vi "MovCorrFuncs.vi"(7 "MovCorrFunc":T5(ring), 11 "Image":T3(plugin-control)) -> (3 "Reference Screen":T3(plugin-control))   [LabVIEW 2020]
uses:
  <vilib>/vision/Image Controls.llb/IMAQ Image.ctl
  <vilib>/vision/NI_Vision_Development_Module.lvlib
panel:
  out "Lines":T1(array[cluster]) {"End Point"."Y" format="%.2f"; "End Point"."X" format="%.2f"; "Start Point"."Y" format="%.2f"; "Start Point"."X" format="%.2f"}
  out "Number of Matches Returned":i32
  out "width":dbl
  out "height":dbl
  out "most Verital":T2
  out "most horizontal":T2
  out "got copy":bool=TRUE
  in  "LUT1":cluster{u16, u16}(slide)={0, 4095} caption="Slide" scale=0.0..4095.0
  out "Reference Rectangles":dbl[][](array[numeric]) format="%.2f"
  out "upper":u16
  out "lower":u16
  out "Number \nof Particles":i32
  out "Mean Value":sgl format="%.2f"
  out "Histogram Graph":T4 {"Incremental Value" format="%.2f"; "Starting Value" format="%.2f"}
  out "temp copy":T3
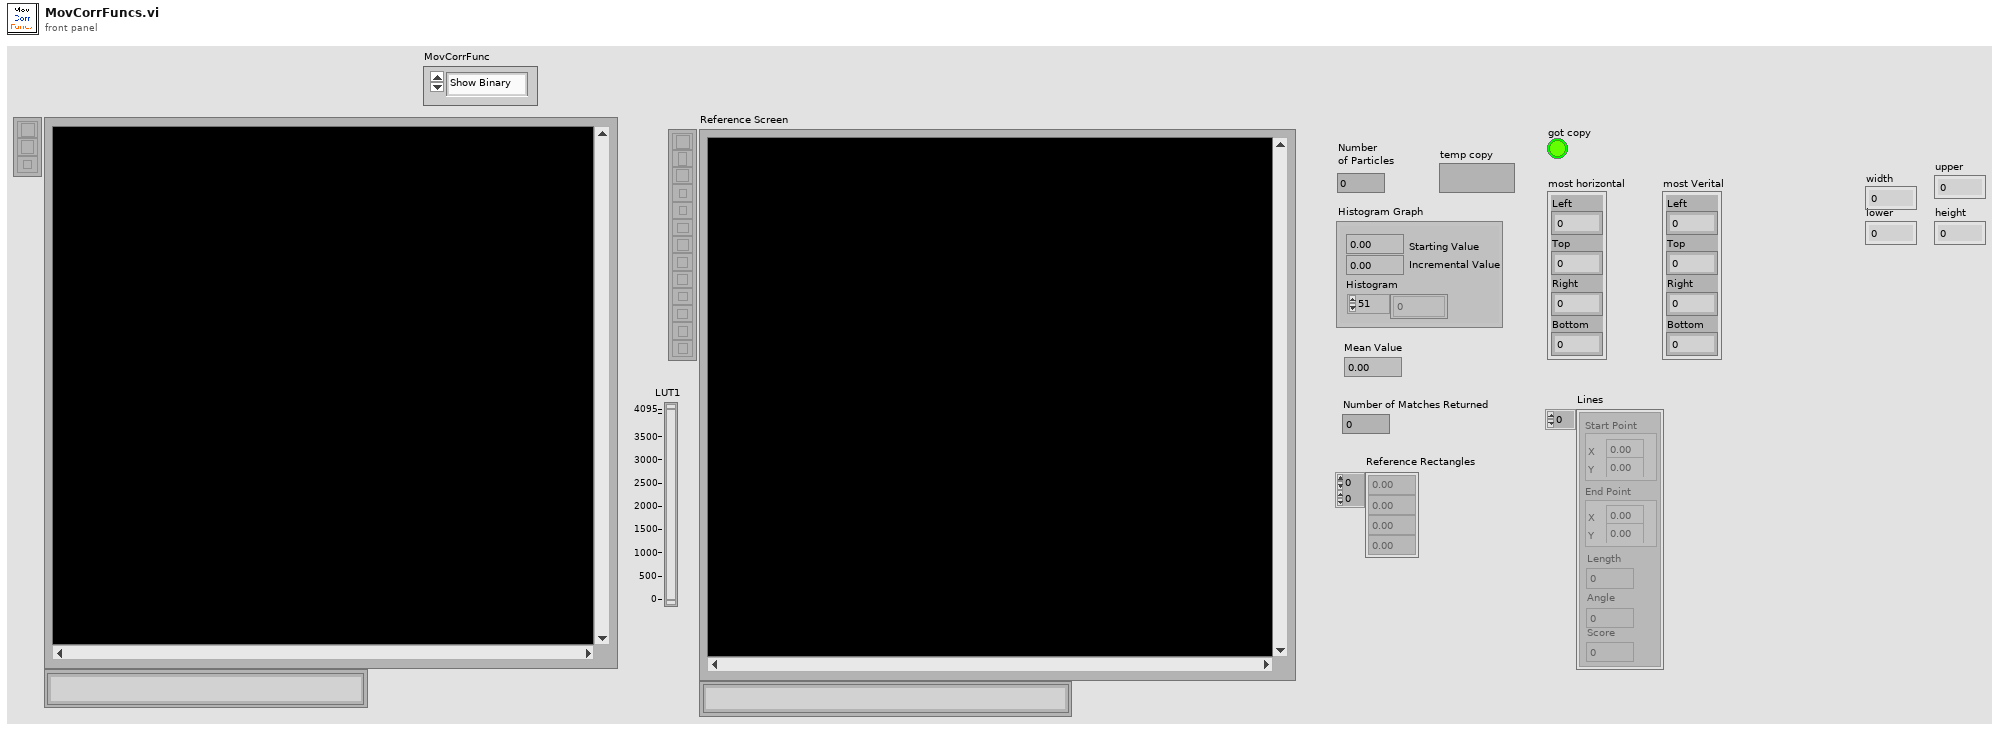
[diagram p1: front panel]
types:
  T1 = cluster{"Start Point":cluster{"X":sgl, "Y":sgl}, "End Point":cluster{"X":sgl, "Y":sgl}, "Length":dbl, "Angle":dbl, "Score":dbl}[]
  T2 = cluster{"Left":i32, "Top":i32, "Right":i32, "Bottom":i32}
  T3 = typedef "IMAQ Image.ctl" = refnum<image>
  T4 = cluster{"Starting Value":sgl, "Incremental Value":sgl, "Histogram":u32[]}
  T5 = enum16{"Show Binary", "Show Dendrite", "Find Lines"}
  T6 = enum32{"AutoM", "Close", "Dilate", "Erode", "Gradient", "Gradient out", "Gradient in", "Hit miss", "Open", "PClose", "POpen", "Thick", "Thin"}
  T7 = typedef "Particle Parameters" = i32
  T8 = typedef "Image Type" = u32
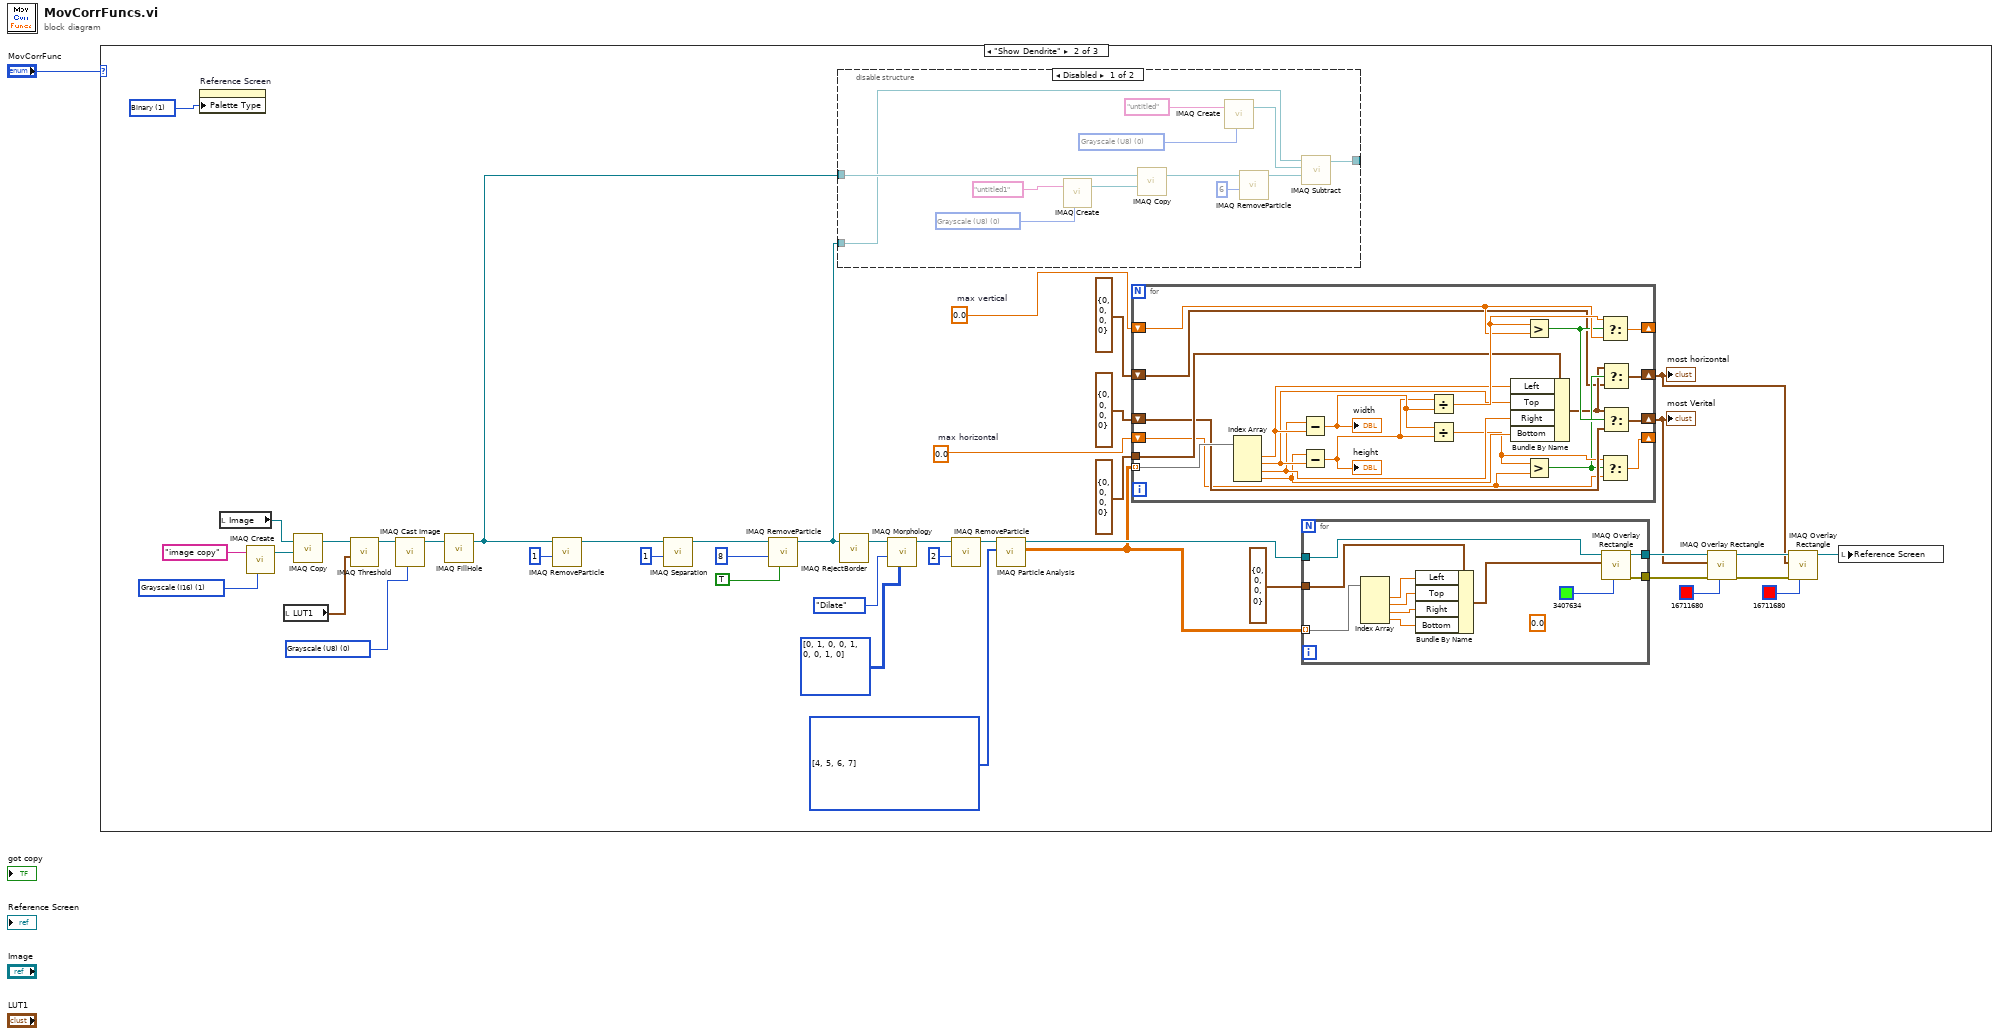
[diagram p0: block diagram]
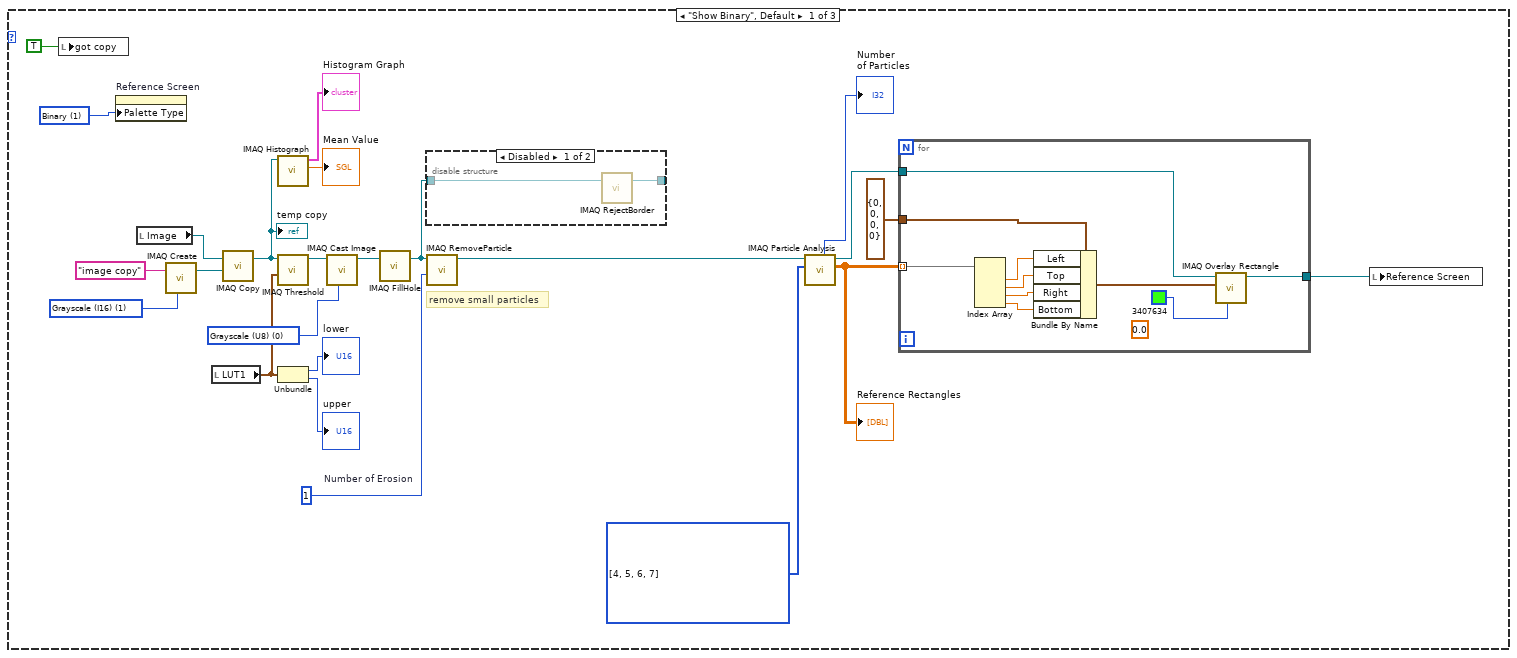
[diagram p2: hidden frame]
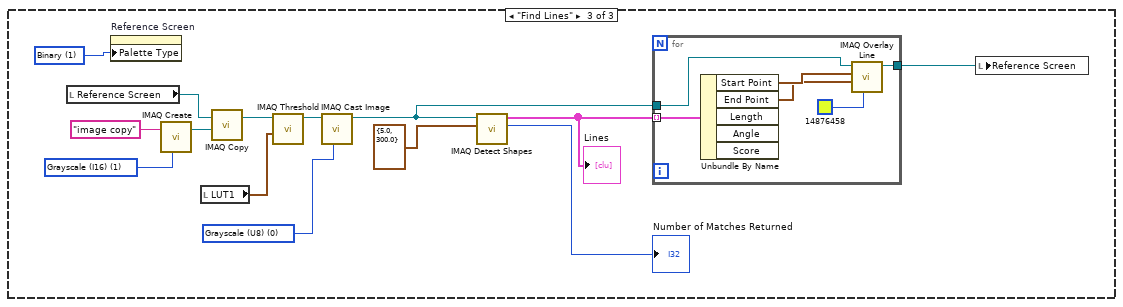
[diagram p5: hidden frame]
diagram:
  n1 = case shown="\"Show Dendrite\"" "MovCorrFunc" {
    frame "Show Binary", Default {
      w3 = u32 1 items=["Grayscale", "Binary", "Gradient", "Rainbow", "Temperature", "User Defined"] ("Palette:Palette Type")
      w12 = T7[] [4, 5, 6, 7] items=["Center of Mass X", "Center of Mass Y", "First Pixel X", "First Pixel Y", "Bounding Rect Left", "Bounding Rect Top", "Bounding Rect Right", "Bounding Rect Bottom", "Max Feret Diameter Start X", "Max Feret Diameter Start Y", "Max Feret Diameter End X", "Max Feret Diameter End Y", "Max Horiz. Segment Length Left", "Max Horiz. Segment Length Right", "Max Horiz. Segment Length Row", "-", "Bounding Rect Width", "Bounding Rect Height", "Bounding Rect Diagonal", "Perimeter", "Convex Hull Perimeter", "Holes' Perimeter", "Max Feret Diameter", "Equivalent Ellipse Major Axis", "Equivalent Ellipse Minor Axis", "Equivalent Ellipse Minor Axis (Feret)", "Equivalent Rect Long Side", "Equivalent Rect Short Side", "Equivalent Rect Diagonal", "Equivalent Rect Short Side (Feret)", "Average Horiz. Segment Length", "Average Vert. Segment Length", "Hydraulic Radius", "Waddel Disk Diameter", "-", "Area", "Holes' Area", "Particle & Holes' Area", "Convex Hull Area", "Image Area", "-", "Number of Holes", "Number of Horiz. Segments", "Number of Vert. Segments", "-", "Orientation", "Max Feret Diameter Orientation", "-", "% Area/Image Area", "% Area/(Particle & Holes' Area)", "Ratio of Equivalent Ellipse Axes", "Ratio of Equivalent Rect Sides", "-", "Elongation Factor", "Compactness Factor", "Heywood Circularity Factor", "Type Factor", "-", "Sum X", "Sum Y", "Sum XX", "Sum XY", "Sum YY", "Sum XXX", "Sum XXY", "Sum XYY", "Sum YYY", "-", "Moment of Inertia XX", "Moment of Inertia XY", "Moment of Inertia YY", "Moment of Inertia XXX", "Moment of Inertia XXY", "Moment of Inertia XYY", "Moment of Inertia YYY", "Norm. Moment of Inertia XX", "Norm. Moment of Inertia XY", "Norm. Moment of Inertia YY", "Norm. Moment of Inertia XXX", "Norm. Moment of Inertia XXY", "Norm. Moment of Inertia XYY", "Norm. Moment of Inertia YYY", "Hu Moment 1", "Hu Moment 2", "Hu Moment 3", "Hu Moment 4", "Hu Moment 5", "Hu Moment 6", "Hu Moment 7"] ("Pixel Measurements")
      w13 = 1  # Number of Erosion
      w15 = T8 0 items=["Grayscale (U8)", "Grayscale (I16)", "Grayscale (SGL)", "Complex (CSG)", "RGB (U32)", "HSL (U32)", "RGB (U64)", "Grayscale (U16)"] ("Image Type")
      w24 = T8 1 items=["Grayscale (U8)", "Grayscale (I16)", "Grayscale (SGL)", "Complex (CSG)", "RGB (U32)", "HSL (U32)", "RGB (U64)", "Grayscale (U16)"] ("Image Type")
      # "remove small particles"
      n2 = local write "got copy"(TRUE) -> ()
      n3 = property on="Reference Screen" class="ImageControl"("Palette Type"=w3) -> ()  [unwired: 2 in, 2 out]
      n4 = local read "Image"() -> (w19:T3)
      n5 = call "IMAQ Create"("Image Name"="image copy", "Image Type"=w24) -> ("New Image"=w23:T3)  [unwired: 3 in, 1 out]
      n6 = local read "LUT1"() -> (w14:cluster{u16, u16})
      n7 = call "IMAQ Copy"("Image Dst"=w23, "Image Src"=w19) -> ("Image Dst Out"=w18:T3)  [unwired: 4 in, 1 out]
      "temp copy" <- w18
      n8 = call "IMAQ Histograph"("Image"=w18) -> ("Mean Value"=→"Mean Value":sgl, "Histogram Graph"=→"Histogram Graph":T4)  [unwired: 7 in, 2 out]
      n9 = call "IMAQ Threshold"("Range"=w14, "Image Src"=w18) -> ("Image Dst Out"=w17:T3)  [unwired: 4 in, 5 out]
      n10 = Unbundle(w14) -> (→"lower":u16, →"upper":u16)
      n11 = call "IMAQ Cast Image"("Image Type"=w15, "Image Src"=w17) -> ("Image Dst Out"=w16:T3)  [unwired: 8 in, 1 out]
      n12 = call "IMAQ FillHole"("Image Src"=w16) -> ("Image Dst Out"=w2:T3)  [unwired: 3 in, 3 out]
      n13 = disable-structure shown="Disabled" {
        disable-tunnel: w2 -> [w27 _]
        disable-tunnel: [w26 _] -> _
        frame Disabled {
          n14 = call "IMAQ RejectBorder"("Image Src"=w27) -> ("Image Dst Out"=w26:T3)  [unwired: 3 in, 3 out]
        }
        frame Enabled {
        }
      }
      n15 = call "IMAQ RemoveParticle"("Number of Erosion"=w13, "Image Src"=w2) -> ("Image Dst Out"=w9:T3)  [unwired: 5 in, 4 out]
      n16 = call "IMAQ Particle Analysis"("Pixel Measurements"=w12, "Image"=w9) -> ("Particle Measurements (Pixels)"=w4:dbl[][], "Image Out (duplicate)"=w11:T3, "Number of Particles"=→"Number \nof Particles":i32)  [unwired: 4 in, 3 out]
      "Reference Rectangles" <- w4
      n17 = for {
        tunnel: [w28] -> w5
        tunnel: w11 -> [w36]
        tunnel: w4 -> [w34] mode=indexing
        tunnel: T2 {"Left"=0, "Top"=0, "Right"=0, "Bottom"=0} ("Rectangle") -> [w35]
        (unwired) 0.0 ("Rotation")
        n18 = Index Array(array=w34) -> (element #1=w32:dbl, element #2=w31:dbl, element #3=w30:dbl, element #4=w29:dbl)  [unwired: 4 in]
        n19 = Bundle By Name(cluster=w35, "Left"=w32, "Top"=w31, "Right"=w30, "Bottom"=w29) -> (w33:T2)
        n20 = call "IMAQ Overlay Rectangle"("Color"=u32 3407634 ("Text Color (black)"), "Rectangle"=w33, "Image"=w36) -> ("Image Out"=w28:T3)  [unwired: 7 in, 1 out]
      }
      n21 = local write "Reference Screen"(w5) -> ()
    }
    frame "Show Dendrite" {
      w53 = 0.0  # max horizontal
      w54 = 0.0  # max vertical
      w70 = T7[] [4, 5, 6, 7] items=["Center of Mass X", "Center of Mass Y", "First Pixel X", "First Pixel Y", "Bounding Rect Left", "Bounding Rect Top", "Bounding Rect Right", "Bounding Rect Bottom", "Max Feret Diameter Start X", "Max Feret Diameter Start Y", "Max Feret Diameter End X", "Max Feret Diameter End Y", "Max Horiz. Segment Length Left", "Max Horiz. Segment Length Right", "Max Horiz. Segment Length Row", "-", "Bounding Rect Width", "Bounding Rect Height", "Bounding Rect Diagonal", "Perimeter", "Convex Hull Perimeter", "Holes' Perimeter", "Max Feret Diameter", "Equivalent Ellipse Major Axis", "Equivalent Ellipse Minor Axis", "Equivalent Ellipse Minor Axis (Feret)", "Equivalent Rect Long Side", "Equivalent Rect Short Side", "Equivalent Rect Diagonal", "Equivalent Rect Short Side (Feret)", "Average Horiz. Segment Length", "Average Vert. Segment Length", "Hydraulic Radius", "Waddel Disk Diameter", "-", "Area", "Holes' Area", "Particle & Holes' Area", "Convex Hull Area", "Image Area", "-", "Number of Holes", "Number of Horiz. Segments", "Number of Vert. Segments", "-", "Orientation", "Max Feret Diameter Orientation", "-", "% Area/Image Area", "% Area/(Particle & Holes' Area)", "Ratio of Equivalent Ellipse Axes", "Ratio of Equivalent Rect Sides", "-", "Elongation Factor", "Compactness Factor", "Heywood Circularity Factor", "Type Factor", "-", "Sum X", "Sum Y", "Sum XX", "Sum XY", "Sum YY", "Sum XXX", "Sum XXY", "Sum XYY", "Sum YYY", "-", "Moment of Inertia XX", "Moment of Inertia XY", "Moment of Inertia YY", "Moment of Inertia XXX", "Moment of Inertia XXY", "Moment of Inertia XYY", "Moment of Inertia YYY", "Norm. Moment of Inertia XX", "Norm. Moment of Inertia XY", "Norm. Moment of Inertia YY", "Norm. Moment of Inertia XXX", "Norm. Moment of Inertia XXY", "Norm. Moment of Inertia XYY", "Norm. Moment of Inertia YYY", "Hu Moment 1", "Hu Moment 2", "Hu Moment 3", "Hu Moment 4", "Hu Moment 5", "Hu Moment 6", "Hu Moment 7"] ("Pixel Measurements")
      w72 = T8 0 items=["Grayscale (U8)", "Grayscale (I16)", "Grayscale (SGL)", "Complex (CSG)", "RGB (U32)", "HSL (U32)", "RGB (U64)", "Grayscale (U16)"] ("Image Type")
      w73 = u32 1 items=["Grayscale", "Binary", "Gradient", "Rainbow", "Temperature", "User Defined"] ("Palette:Palette Type")
      w78 = T8 1 items=["Grayscale (U8)", "Grayscale (I16)", "Grayscale (SGL)", "Complex (CSG)", "RGB (U32)", "HSL (U32)", "RGB (U64)", "Grayscale (U16)"] ("Image Type")
      n22 = property on="Reference Screen" class="ImageControl"("Palette Type"=w73) -> ()  [unwired: 2 in, 2 out]
      n23 = local read "Image"() -> (w76:T3)
      n24 = call "IMAQ Create"("Image Name"="image copy", "Image Type"=w78) -> ("New Image"=w77:T3)  [unwired: 3 in, 1 out]
      n25 = local read "LUT1"() -> (w74:cluster{u16, u16})
      n26 = call "IMAQ Copy"("Image Dst"=w77, "Image Src"=w76) -> ("Image Dst Out"=w75:T3)  [unwired: 4 in, 1 out]
      n27 = call "IMAQ Threshold"("Range"=w74, "Image Src"=w75) -> ("Image Dst Out"=w40:T3)  [unwired: 4 in, 5 out]
      n28 = call "IMAQ Cast Image"("Image Type"=w72, "Image Src"=w40) -> ("Image Dst Out"=w39:T3)  [unwired: 8 in, 1 out]
      n29 = call "IMAQ FillHole"("Image Src"=w39) -> ("Image Dst Out"=w38:T3)  [unwired: 5 in, 1 out]
      n30 = call "IMAQ RemoveParticle"("Number of Erosion"=1, "Image Src"=w38) -> ("Image Dst Out"=w67:T3)  [unwired: 5 in, 4 out]
      n31 = call "IMAQ Separation"("Nb of Erosion"=1, "Image Src"=w67) -> ("Image Dst Out"=w64:T3)  [unwired: 8 in, 1 out]
      n32 = call "IMAQ RemoveParticle"("Low Pass/High Pass (Low)"=TRUE, "Number of Erosion"=8, "Image Src"=w64) -> ("Image Dst Out"=w62:T3)  [unwired: 4 in, 4 out]
      n33 = disable-structure shown="Disabled" {
        disable-tunnel: w38 -> [w112 _]
        disable-tunnel: w62 -> [w111 _]
        disable-tunnel: [w110 _] -> _
        frame Disabled {
          w103 = T8 0 items=["Grayscale (U8)", "Grayscale (I16)", "Grayscale (SGL)", "Complex (CSG)", "RGB (U32)", "HSL (U32)", "RGB (U64)", "Grayscale (U16)"] ("Image Type")
          w108 = T8 0 items=["Grayscale (U8)", "Grayscale (I16)", "Grayscale (SGL)", "Complex (CSG)", "RGB (U32)", "HSL (U32)", "RGB (U64)", "Grayscale (U16)"] ("Image Type")
          n34 = call "IMAQ Create"("Image Name"="untitled1", "Image Type"=w103) -> ("New Image"=w102:T3)  [unwired: 3 in, 1 out]
          n35 = call "IMAQ Copy"("Image Dst"=w102, "Image Src"=w112) -> ("Image Dst Out"=w101:T3)  [unwired: 4 in, 1 out]
          n36 = call "IMAQ Create"("Image Name"="untitled", "Image Type"=w108) -> ("New Image"=w106:T3)  [unwired: 3 in, 1 out]
          n37 = call "IMAQ RemoveParticle"("Number of Erosion"=6, "Image Src"=w101) -> ("Image Dst Out"=w105:T3)  [unwired: 5 in, 4 out]
          n38 = call "IMAQ Subtract"("Image Src A"=w111, "Image Dst"=w106, "Image Src B"=w105) -> ("Image Dst Out"=w110:T3)  [unwired: 4 in, 1 out]
        }
        frame Enabled {
        }
      }
      n39 = call "IMAQ RejectBorder"("Image Src"=w62) -> ("Image Dst Out"=w60:T3)  [unwired: 5 in, 1 out]
      n40 = call "IMAQ Morphology"("Structuring Element"=i32[][] [[0, 1, 0], [0, 1, 0], [0, 1, 0]], "Operation"=T6."Dilate", "Image Src"=w60) -> ("Image Dst Out"=w57:T3)  [unwired: 7 in, 1 out]
      n41 = call "IMAQ RemoveParticle"("Number of Erosion"=2, "Image Src"=w57) -> ("Image Dst Out"=w56:T3)  [unwired: 5 in, 4 out]
      n42 = call "IMAQ Particle Analysis"("Pixel Measurements"=w70, "Image"=w56) -> ("Particle Measurements (Pixels)"=w55:dbl[][], "Image Out (duplicate)"=w69:T3)  [unwired: 4 in, 4 out]
      n43 = for {
        tunnel: w55 -> [w100] mode=indexing
        shift-right: [w95] -> _
        shift-left: w54 -> [w96]
        shift-right: [w84] -> _
        shift-left: w53 -> [w85]
        tunnel: T2 {"Left"=0, "Top"=0, "Right"=0, "Bottom"=0} ("Rectangle") -> [w90]
        shift-right: [w88] -> w48
        shift-left: T2 {"Left"=0, "Top"=0, "Right"=0, "Bottom"=0} ("Rectangle") -> [w87]
        shift-right: [w81] -> w45
        shift-left: T2 {"Left"=0, "Top"=0, "Right"=0, "Bottom"=0} ("Rectangle") -> [w80]
        n44 = Index Array(array=w100) -> (element #1=w94:dbl, element #2=w93:dbl, element #3=w92:dbl, element #4=w91:dbl)  [unwired: 4 in]
        n45 = Subtract(x=w92, y=w94) -> (x-y=w99:dbl)
        "width" <- w99
        n46 = Subtract(x=w91, y=w93) -> (x-y=w98:dbl)
        "height" <- w98
        n47 = Divide(x=w98, y=w99) -> (x/y=w97:dbl)
        n48 = Divide(x=w99, y=w98) -> (x/y=w86:dbl)
        n49 = Bundle By Name(cluster=w90, "Left"=w94, "Top"=w93, "Right"=w92, "Bottom"=w91) -> (w82:T2)
        n50 = Greater?(x=w97, y=w96) -> (0:w89:bool)
        n51 = Greater?(x=w86, y=w85) -> (0:w83:bool)
        n52 = Select(t=w97, s=w89, f=w96) -> (s? t:f=w95:dbl)
        n53 = Select(t=w86, s=w83, f=w85) -> (s? t:f=w84:dbl)
        n54 = Select(t=w82, s=w83, f=w80) -> (s? t:f=w81:T2)
        n55 = Select(t=w82, s=w89, f=w87) -> (s? t:f=w88:T2)
      }
      "most Verital" <- w48
      "most horizontal" <- w45
      n56 = for {
        tunnel: [w114] -> w49
        tunnel: w69 -> [w122]
        tunnel: w55 -> [w120] mode=indexing
        tunnel: T2 {"Left"=0, "Top"=0, "Right"=0, "Bottom"=0} ("Rectangle") -> [w121]
        tunnel: [w113] -> w42
        (unwired) 0.0 ("Rotation")
        n57 = Index Array(array=w120) -> (element #1=w118:dbl, element #2=w117:dbl, element #3=w116:dbl, element #4=w115:dbl)  [unwired: 4 in]
        n58 = Bundle By Name(cluster=w121, "Left"=w118, "Top"=w117, "Right"=w116, "Bottom"=w115) -> (w119:T2)
        n59 = call "IMAQ Overlay Rectangle"("Color"=u32 3407634 ("Text Color (black)"), "Rectangle"=w119, "Image"=w122) -> ("error out"=w113:errorcluster, "Image Out"=w114:T3)  [unwired: 7 in]
      }
      n60 = call "IMAQ Overlay Rectangle"("Color"=u32 16711680, "error in (no error)"=w42, "Rectangle"=w48, "Image"=w49) -> ("error out"=w41:errorcluster, "Image Out"=w46:T3)  [unwired: 6 in]
      n61 = call "IMAQ Overlay Rectangle"("Color"=u32 16711680, "error in (no error)"=w41, "Rectangle"=w45, "Image"=w46) -> ("Image Out"=w43:T3)  [unwired: 6 in, 1 out]
      n62 = local write "Reference Screen"(w43) -> ()
    }
    frame "Find Lines" {
      w129 = u32 1 items=["Grayscale", "Binary", "Gradient", "Rainbow", "Temperature", "User Defined"] ("Palette:Palette Type")
      w130 = T8 0 items=["Grayscale (U8)", "Grayscale (I16)", "Grayscale (SGL)", "Complex (CSG)", "RGB (U32)", "HSL (U32)", "RGB (U64)", "Grayscale (U16)"] ("Image Type")
      w136 = T8 1 items=["Grayscale (U8)", "Grayscale (I16)", "Grayscale (SGL)", "Complex (CSG)", "RGB (U32)", "HSL (U32)", "RGB (U64)", "Grayscale (U16)"] ("Image Type")
      n63 = local read "Reference Screen"() -> (w134:T3)
      n64 = property on="Reference Screen" class="ImageControl"("Palette Type"=w129) -> ()  [unwired: 2 in, 2 out]
      n65 = call "IMAQ Create"("Image Name"="image copy", "Image Type"=w136) -> ("New Image"=w135:T3)  [unwired: 3 in, 1 out]
      n66 = local read "LUT1"() -> (w131:cluster{u16, u16})
      n67 = call "IMAQ Copy"("Image Dst"=w135, "Image Src"=w134) -> ("Image Dst Out"=w132:T3)  [unwired: 4 in, 1 out]
      n68 = call "IMAQ Threshold"("Range"=w131, "Image Src"=w132) -> ("Image Dst Out"=w133:T3)  [unwired: 4 in, 5 out]
      n69 = call "IMAQ Cast Image"("Image Type"=w130, "Image Src"=w133) -> ("Image Dst Out"=w125:T3)  [unwired: 8 in, 1 out]
      n70 = call-poly "IMAQ Detect Shapes"("Line Descriptor"=cluster{"Min Length":dbl, "Max Length":dbl} {"Min Length"=5.0, "Max Length"=300.0}, "Image"=w125) -> ("Number of Matches Returned"=→"Number of Matches Returned":i32, "Lines"=w126:T1)  [unwired: 7 in, 1 out]
      "Lines" <- w126
      n71 = for {
        tunnel: w126 -> [w143] mode=indexing
        tunnel: w125 -> [w142]
        tunnel: [w138] -> w124
        n72 = Unbundle By Name(w143) -> ("Start Point"=w141:cluster{"X":sgl, "Y":sgl}, "End Point"=w140:cluster{"X":sgl, "Y":sgl})  [unwired: 3 out]
        n73 = call "IMAQ Overlay Line"("Color"=u32 14876458, "End Point"=w140, "Start Point"=w141, "Image"=w142) -> ("Image Out"=w138:T3)  [unwired: 6 in, 1 out]
      }
      n74 = local write "Reference Screen"(w124) -> ()
    }
  }
